vi "Display.vi"(8 "error in":errorcluster, 11 "Timeout One Button in":refnum<class "Gif - Timeout One Button.lvclass">) -> (0 "error out":errorcluster, 3 "Timeout One Button out":refnum<class "Gif - Timeout One Button.lvclass">)   [LabVIEW 2021, in "Pop-Up.lvlib" / "Gif - Timeout One Button.lvclass"]
doc: "This vi displays the custom image one button timeout popup.\n\n<b>Code Developed By:</b>\nDaniel Coons\nTechnology Service Corporation\n1983 S Liberty Drive\nBloomington, IN 47403\nPhone: 812 558-7100\ndaniel.coons@tsc.com\nwww.tsc.com/atcs"
uses:
  Gif - Timeout One Button.lvclass
  C:/Development/TSC.Pop-Up/Popup/Popup.lvclass
  C:/Development/TSC.Pop-Up/Gif/Gif Parent.lvclass
  Gif - Timeout One Button.lvclass/Gif - Timeout One Button.ctl
  Popup/Popup.lvclass/Popup.ctl
  Gif Parent.lvclass/Gif Parent.ctl
  Popup/Data Member Access/Read Theme.vi
  Read Delays.vi
  Read Gif Images.vi
  Theme/Theme.lvclass
  Popup/Popup.lvclass
  user32.dll
  C:/Development/TSC.Pop-Up/Gif/Custom/Gif - Timeout One Button/Gif - Timeout One Button.lvclass
panel:
  in  "closer":bool
  out "header":bool
  out "count":string
  in  "OK":bool
  out "Message":string
  out "2D Picture":picture
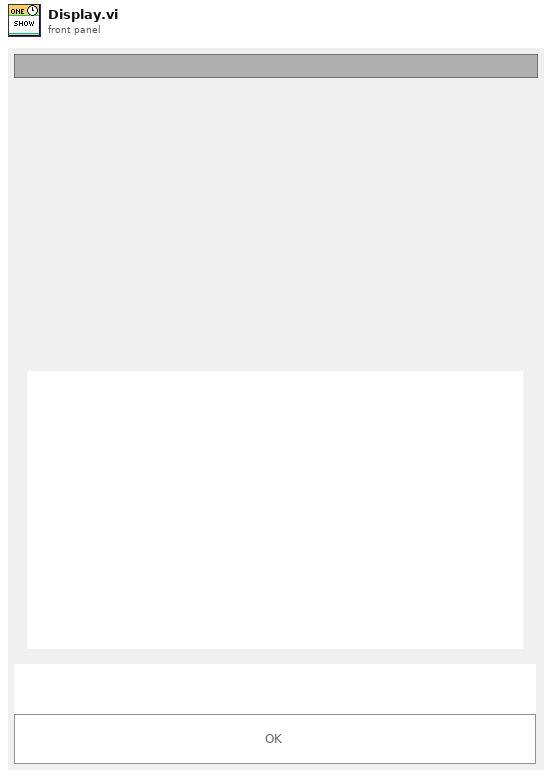
[diagram p1: front panel]
types:
  T1 = typedef "LVPoint32TypeDef.ctl" = cluster{"Horizontal":i32, "Vertical":i32}
  T2 = typedef "LVPositionTypeDef.ctl" = cluster{"Left":i32, "Top":i32}
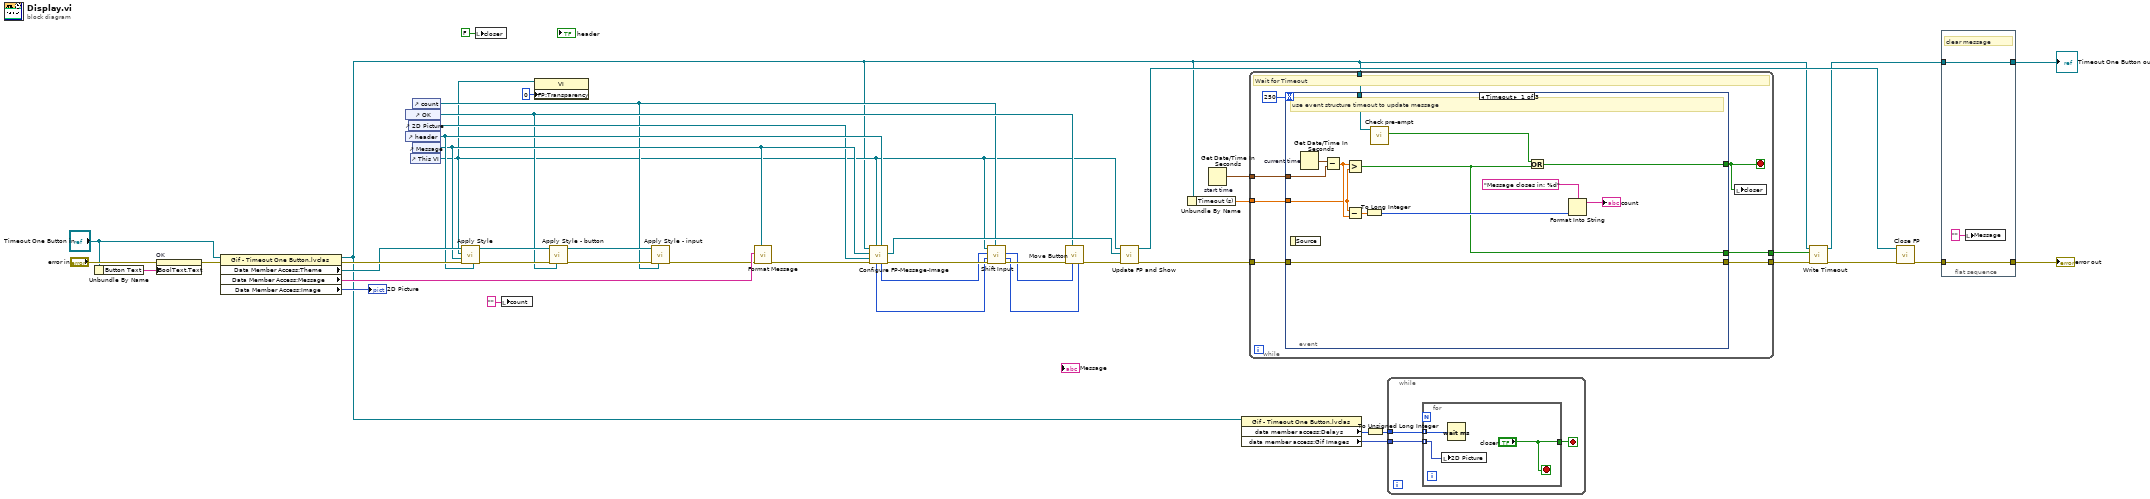
[diagram p0: block diagram]
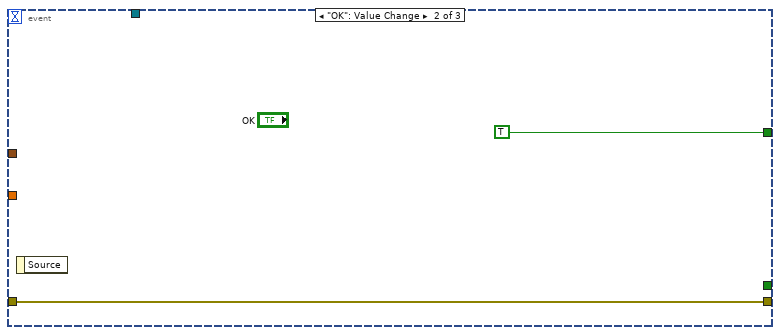
[diagram p2: hidden frame]
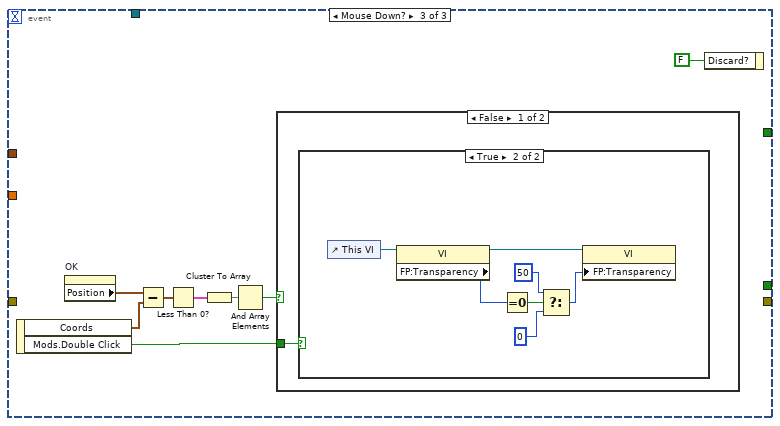
[diagram p3: hidden frame]
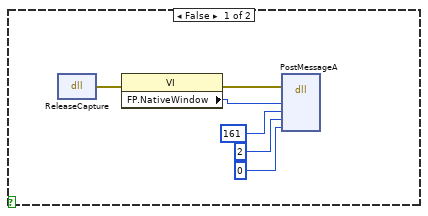
[diagram p4: hidden frame]
diagram:
  n1 = Unbundle By Name("Timeout One Button in") -> ("Button Text"=w42:string)
  n2 = property on="OK" class="Bool"(error in="error in", "BoolText.Text"=w42) -> (error out=w44:errorcluster)  [unwired: 1 in, 1 out]
  n3 = property class="Gif - Timeout One Button.lvclas"(reference="Timeout One Button in", error in=w44) -> (reference out=w3:refnum<class "Gif - Timeout One Button.lvclass">, error out=w30:errorcluster, "Data Member Access:Theme"=w29:refnum<class "Theme.lvclass">, "Data Member Access:Message"=w27:string, "Data Member Access:Image"=→"2D Picture":picture)
  n4 = control-ref of="OK"() -> (w20:refnum<vi>)
  n5 = control-ref of="header"() -> (w25:refnum<vi>)
  n6 = control-ref of="2D Picture"() -> (w23:refnum<vi>)
  n7 = control-ref of="This VI"() -> (w10:refnum<vi>)
  n8 = control-ref of="count"() -> (w15:refnum<vi>)
  n9 = control-ref of="Message"() -> (w24:refnum<vi>)
  n10 = call "Apply Style.vi"("header ref"=w25, "error in (no error)"=w30, "message ref"=w24, "pop up ref"=w10, "Theme in"=w29) -> ("error out"=w32:errorcluster, "Theme out"=w31:refnum<class "Theme.lvclass">)  [unwired: 5 in]
  n11 = local write "closer"(FALSE ("closer")) -> ()
  n12 = local write "count"("" ("count")) -> ()
  n13 = property class="VI"(reference=w10, "FP:Transparency"=u8 0 ("Front Panel Window:Transparency")) -> ()  [unwired: 1 in, 2 out]
  n14 = call "Apply Style - button.vi"("button ref"=w20, "error in (no error)"=w32, "Theme in"=w31) -> ("error out"=w28:errorcluster, "Theme out"=w17:refnum<class "Theme.lvclass">)  [unwired: 7 in]
  n15 = call "Apply Style - input.vi"("input ref"=w15, "error in (no error)"=w28, "Theme in"=w17) -> ("error out"=w18:errorcluster)  [unwired: 7 in, 1 out]
  n16 = call "Format Message.vi"("formatted string"=w24, "error in"=w18, "String Input"=w27) -> ("error out"=w26:errorcluster)  [unwired: 7 in, 1 out]
  n17 = call "Configure FP-Message-Image.vi"("header ref"=w25, "Pop Up ref"=w10, "error in (no error)"=w26, "Image ref"=w23, "Message ref"=w24, "Popup in"=w3) -> ("error out"=w22:errorcluster, "Panel Ref"=w21:refnum<vi>, "Panel Width"=w14:i32, "Panel Height"=w12:i32)  [unwired: 1 in, 1 out]
  n18 = call "Shift Input.vi"("Control"=w15, "Error In"=w22, "Panel Height"=w12, "Panel Width"=w14, "Pop Up ref"=w10) -> ("Error Out"=w16:errorcluster, "Panel Height out"=w11:i32, "Panel Width out"=w13:i32)  [unwired: 4 in]
  n19 = call "Move Button.vi"("Panel Height"=w11, "Panel Width"=w13, "Button"=w20, "Error In"=w16) -> ("Error Out"=w19:errorcluster)  [unwired: 6 in, 1 out]
  n20 = call "Update FP and Show.vi"("error in (no error)"=w19, "Panel Ref"=w21, "VI in"=w10) -> ("error out"=w40:errorcluster, "VI out"=w36:refnum<vi>)  [unwired: 7 in]
  n21 = Unbundle By Name(w3) -> ("Timeout (s)"=w35:dbl)
  n22 = Get Date/Time In Seconds "start time"() -> (seconds since 1Jan1904=w34:timestamp)
  n23 = property class="Gif - Timeout One Button.lvclas"(reference=w3) -> ("data member access:Delays"=w8:i32[], "data member access:Gif Images"=w7:picture[])  [unwired: 1 in, 2 out]
  n24 = while {
    tunnel: [w50] -> w41
    tunnel: w40 -> [w51]
    tunnel: w34 -> [w54]
    tunnel: w35 -> [w53]
    tunnel: w3 -> [w49]
    tunnel: [w47] -> w1
    stop <- w48 stop-if-true
    # "Wait for Timeout"
    n25 = event shown="[0] Timeout" {
      selector: _ -> [_ _ _]
      dyn-events: _ -> [_ _ _]
      timeout: 250 -> [_ _ _]
      tunnel: w54 -> [w67 _ _]
      tunnel: [w58 TRUE _] -> w48
      tunnel: w53 -> [w63 _ _]
      tunnel: w51 -> [w60 w68 _]
      tunnel: [w60 w68 _] -> w50
      tunnel: w49 -> [w59 _ _]
      tunnel: [w55 _ _] -> w47
      event Timeout {
        # "use event structure timeout to update message"
        n26 = event-data() -> ()  [unwired: 1 in, 1 out]
        n27 = Get Date/Time In Seconds "current time"() -> (seconds since 1Jan1904=w66:timestamp)
        n28 = Subtract(x=w66, y=w67) -> (x-y=w65:dbl)
        n29 = Greater?(x=w65, y=w63) -> (0:w55:bool)
        n30 = Subtract(x=w63, y=w65) -> (x-y=w64:dbl)
        n31 = To Long Integer(number=w64) -> (32bit integer=w61:i32)
        n32 = call "Check pre-empt.vi"("_Popup in"=w59) -> ("Pre-empted?"=w57:bool)  [unwired: 8 in, 2 out]
        n33 = Or(x=w57, y=w55) -> (x .or. y?=w58:bool)
        n34 = Format Into String(format string="Message closes in: %d", w61) -> (resulting string=→"count":string)  [unwired: 2 in, 1 out]
      }
      event "OK": Value Change {
        n35 = event-data() -> ()  [unwired: 1 in, 1 out]
      }
      event Mouse Down? {
        n36 = event-data() -> ("Coords"=w70:T1, "Mods.Double Click"=w71:bool)  [unwired: 1 in]
        n37 = property on="OK" class="Bool"() -> ("Position"=w76:T2)  [unwired: 2 in, 2 out]
        n38 = Subtract(x=w76, y=w70) -> (x-y=w75:T2)
        n39 = Less Than 0?(x=w75) -> (x < 0?=w74:cluster{"Left":bool, "Top":bool})
        n40 = Cluster To Array(cluster=w74) -> (array=w73:bool[])
        n41 = And Array Elements(Boolean array=w73) -> (logical AND=w72:bool)
        n42 = case shown="False" w72 {
          tunnel: w71 -> [w78 _]
          frame False {
            n43 = case shown="True" w78 {
              frame False {
                n44 = dll-call lib="user32.dll" fn="ReleaseCapture"() -> (error out=w82:errorcluster)  [unwired: 4 in, 1 out]
                n45 = property class="VI"(error in=w82) -> (error out=w83:errorcluster, "FP.NativeWindow"=w84:u64)  [unwired: 1 in, 1 out]
                n46 = dll-call lib="user32.dll" fn="PostMessageA"(error in=w83, "hWnd"=w84, "Msg"=161, "wParam"=2, "lParam"=0) -> ()  [unwired: 7 in, 2 out]
              }
              frame True {
                n47 = control-ref of="This VI"() -> (w91:refnum<vi>)
                n48 = property class="VI"(reference=w91) -> (reference out=w89:refnum<vi>, "FP:Transparency"=w90:u8)  [unwired: 1 in, 1 out]
                n49 = Equal To 0?(x=w90) -> (x = 0?=w88:bool)
                n50 = Select(t=u8 50, s=w88, f=u8 0) -> (s? t:f=w87:u8)
                n51 = property class="VI"(reference=w89, "FP:Transparency"=w87) -> ()  [unwired: 1 in, 2 out]
              }
            }
          }
          frame True {
          }
        }
        n52 = event-data("Discard?"=FALSE) -> ()  [unwired: 1 in, 1 out]
      }
    }
    n53 = local write "closer"(w48) -> ()
  }
  n54 = To Unsigned Long Integer(number=w8) -> (unsigned 32bit integer=w6:u32[])
  n55 = while {
    tunnel: w6 -> [w93]
    tunnel: w7 -> [w92]
    stop <- w94 stop-if-true
    n56 = for {
      tunnel: ["closer"] -> w94
      tunnel: w93 -> [w96] mode=indexing
      tunnel: w92 -> [w95] mode=indexing
      stop <- "closer" stop-if-true
      n57 = local write "2D Picture"(w95) -> ()
      n58 = Wait (ms)(milliseconds to wait=w96) -> ()  [unwired: 1 out]
    }
  }
  n59 = call "Write Timeout.vi"("error in (no error)"=w41, "Timeout?"=w1, "Popup in"=w3) -> ("error out"=w4:errorcluster, "Popup out"=w2:refnum<class "Gif - Timeout One Button.lvclass">)  [unwired: 7 in]
  n60 = call "Close FP.vi"("error in (no error)"=w4, "VI in"=w36) -> ("error out"=w39:errorcluster)  [unwired: 9 in]
  n61 = flat-sequence {
    tunnel: w39 -> [w100]
    tunnel: [w100] -> w38
    tunnel: w2 -> [w98]
    tunnel: [w98] -> w37
    frame #0 {
      # "clear message"
      n62 = local write "Message"("" ("Message")) -> ()
    }
  }
  "error out" <- w38
  "Timeout One Button out" <- w37
